vi "ObtainObject.vi"(8 "ErrorIn":errorcluster, 9 "Label":string, 10 "ObjectName":string, 11 "Type":refnum<class "ITAFObject.lvclass">) -> (0 "ErrorOut":errorcluster, 3 "ObjectOut":refnum<class "ITAFObject.lvclass">)   [LabVIEW 2021]
uses:
  Interface_TAF_ITAFObject/ITAFObject/ITAFObject.lvclass
  Interface_TAF_IApplicationConfiguration/IApplicationConfiguration/IApplicationConfiguration.lvclass
  56a36cc8-d42a-406d-9e1b-e03f28116498.vi
  <vilib>/TriekselSoft/TracerLibrary/TracerLibrary/Tracer/protected/SendMessage.vi
  <vilib>/TriekselSoft/TracerLibrary/TracerLibrary/Tracer/protected/Timestamp.vi
  56a36cc8-d42a-406d-9e1b-e03f28116498.vi/f75db090-0877-4668-94fb-75c2140b1617.vi
  <vilib>/TriekselSoft/TracerLibrary/TracerLibrary/Tracer/Tracer_Level-Debug.vi
  <vilib>/JDP Science/JSONtext/Variant to JSON Text.vi
  <vilib>/TriekselSoft/TracerLibrary/TracerLibrary/Tracer/protected/Tracer_ClassAttributes.vi
  <vilib>/JDP Science/JSONtext/LVClass Serializer/JSONtext LVClass Serializer.lvclass
  Application.lvclass/Application.ctl
  Application.lvclass
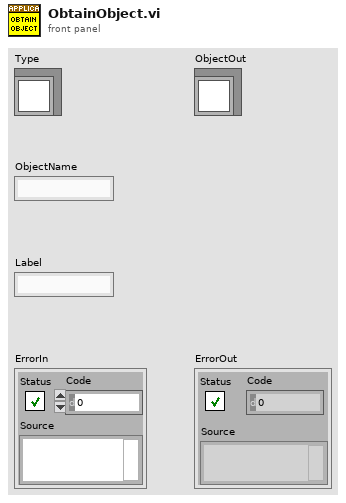
[diagram p1: front panel]
types:
  T1 = cluster{"Label":string, "ObjectName":string, "class name":string}
  T2 = typedef "Application.lvclass/ObjectAttributes.ctl" = cluster{"Objects":variant, "BasePath":path, "Application":refnum<class "Application.lvclass">}
  T3 = typedef "IApplicationConfiguration.lvclass/ObjectData.ctl" = cluster{"Label":string, "ObjectName":string, "Type":string}
  T4 = typedef "IApplicationConfiguration.lvclass/ObjectDataDetails.ctl" = cluster{"ObjectName":string, "ObjectType":string, "Interfaces":T3[]}
  T5 = typedef "ClusterArrayConversion.lvlib/BundledArray.ctl" = cluster{"Label":string, "Object":refnum<class>, "Array":bool}
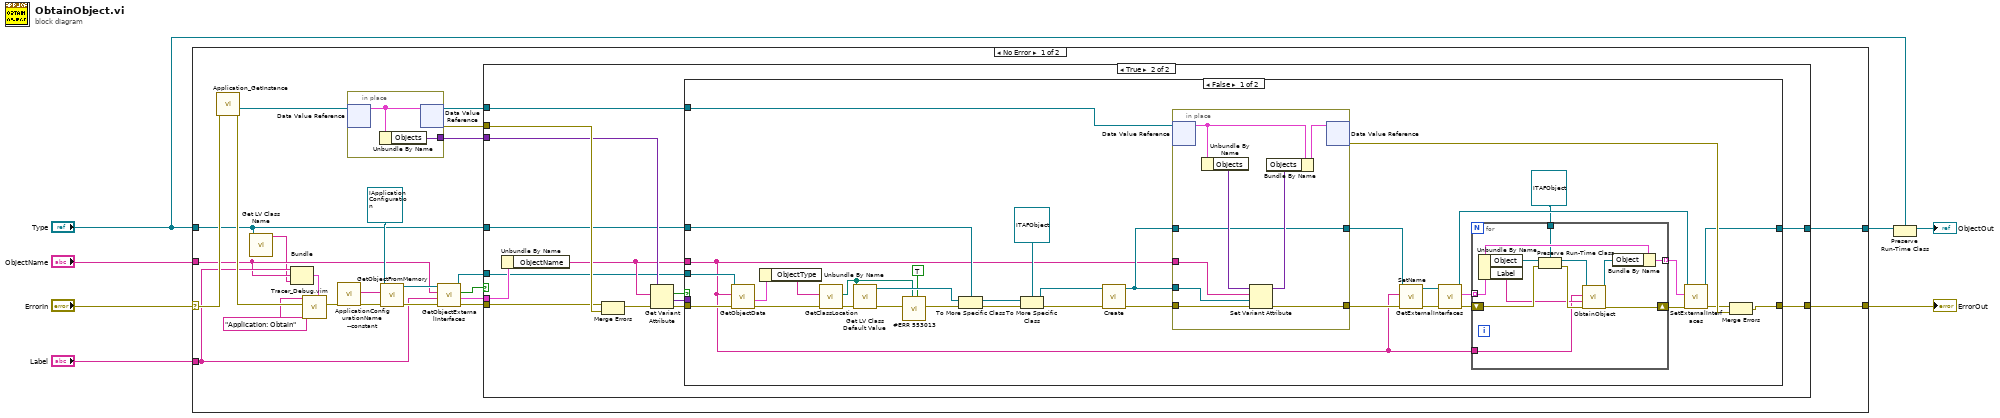
[diagram p0: block diagram]
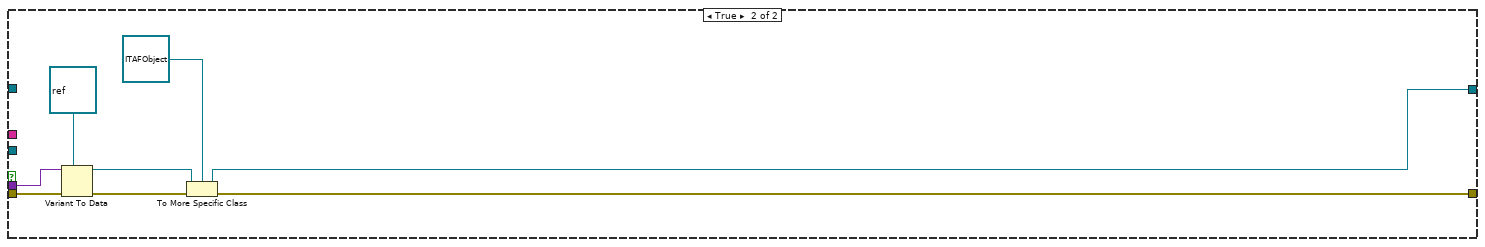
[diagram p3: hidden frame]
diagram:
  n1 = case shown="No Error" "ErrorIn" {
    selector: "ErrorIn" -> [w30 w112]
    tunnel: [w28 w112] -> w6
    tunnel: "ObjectName" -> [w13 _]
    tunnel: "Type" -> [w12 _]
    tunnel: [w23 _] -> w4
    tunnel: "Label" -> [w14 _]
    frame No Error {
      n2 = call "Application_GetInstance.vi"("ErrorIn"=w30) -> ("ErrorOut"=w25:errorcluster, "DVRRefOut"=w22:refnum<data-value>)  [unwired: 6 in, 3 out]
      n3 = call <vilib>:"Get LV Class Name.vi"("object"=w12) -> ("class name"=w11:string)  [unwired: 9 in, 1 out]
      n4 = Bundle("Label"=w14, "ObjectName"=w13, "class name"=w11) -> (w10:T1)  [unwired: 1 in]
      n5 = call "Tracer_Debug.vim"("Data"=w10, "Error In"=w25, "Text"="Application: Obtain") -> ("Error Out"=w24:errorcluster)  [unwired: 8 in]
      n6 = call "ApplicationConfigurationName --constant.vi"() -> ("AppConfigName"=w18:string)  [unwired: 10 in, 1 out]
      n7 = in-place {
        in-place-border: [w110] -> w21
        n8 = in-place-dvr #1(w22) -> (w111:T2)  [unwired: 1 out]
        n9 = Unbundle By Name(w111) -> ("Objects"=w110:variant)
        n10 = in-place-dvr #1(w111) -> (w20:refnum<data-value>, w29:errorcluster)
      }
      n11 = call "GetObjectFromMemory.vi"("ErrorIn"=w24, "ObjectName"=w18, "Type"=refnum<class "IApplicationConfiguration.lvclass"> refnum ("IApplicationStructure")) -> ("ErrorOut"=w27:errorcluster, "ObjectOut"=w17:refnum<class "IApplicationConfiguration.lvclass">)  [unwired: 7 in]
      n12 = call-dynamic "GetObjectExternalInterfaces.vi"("ErrorIn"=w27, "Label"=w14, "ThisObject"=w13, "ObjectIn"=w17) -> ("ErrorOut"=w26:errorcluster, "ObjectData"=w16:T3, "Valid"=w9:bool, "ObjectOut"=w8:refnum<class "IApplicationConfiguration.lvclass">)  [unwired: 4 in]
      n13 = case shown="True" w9 {
        tunnel: [w31 w41] -> w23
        tunnel: w29 -> [_ w46]
        tunnel: w21 -> [_ w38]
        tunnel: w20 -> [_ w37]
        tunnel: [w32 w43] -> w28
        tunnel: w26 -> [w32 w42]
        tunnel: w16 -> [_ w36]
        tunnel: w12 -> [w31 w34]
        tunnel: w8 -> [_ w33]
        frame False {
        }
        frame True {
          n14 = Unbundle By Name(w36) -> ("ObjectName"=w35:string)
          n15 = Merge Errors(w42, w46) -> (w45:errorcluster)
          n16 = Get Variant Attribute(Variant=w38, name=w35, error in=w45) -> (found=w40:bool, value=w39:variant, error out=w44:errorcluster)  [unwired: 1 in, 1 out]
          n17 = case shown="False" w40 {
            tunnel: w44 -> [w69 w109]
            tunnel: w34 -> [w61 _]
            tunnel: [w81 w107] -> w43
            tunnel: [w53 w102] -> w41
            tunnel: w39 -> [_ w105]
            tunnel: w37 -> [w66 _]
            tunnel: w35 -> [w50 _]
            tunnel: w33 -> [w51 _]
            frame False {
              n18 = call-dynamic "GetObjectData.vi"("ErrorIn"=w69, "Object"=w50, "ReferenceIn"=w51) -> ("ErrorOut"=w68:errorcluster, "Object2"=w49:T4)  [unwired: 6 in, 1 out]
              n19 = Unbundle By Name(w49) -> ("ObjectType"=w48:string)
              n20 = call "GetClassLocation.vi"("ErrorIn"=w68, "ClassString"=w48) -> ("ErrorOut"=w67:errorcluster, "ClassFilePath"=w47:path)  [unwired: 8 in]
              n21 = call <vilib>:"Get LV Class Default Value.vi"("error in (no error)"=w67, "class path"=w47) -> ("error out"=w77:errorcluster, "object"=w62:refnum<class>)  [unwired: 8 in]
              n22 = call "#ERR 553013"("MergeErrors"=TRUE, "Data"=w47, "error in (no error)"=w77) -> ("error out"=w75:errorcluster)  [unwired: 8 in]
              n23 = To More Specific Class(target class=w61, reference=w62, error in=w75) -> (specific class reference=w60:refnum<class "ITAFObject.lvclass">, error out=w76:errorcluster)
              n24 = To More Specific Class(target class=refnum<class "ITAFObject.lvclass"> refnum ("ClassActor"), reference=w60, error in=w76) -> (specific class reference=w64:refnum<class "ITAFObject.lvclass">, error out=w79:errorcluster)
              n25 = call-dynamic "Create.vi"("ErrorIn"=w79, "ObjectIn"=w64) -> ("ErrorOut"=w78:errorcluster, "ObjectOut"=w63:refnum<class "ITAFObject.lvclass">)  [unwired: 8 in]
              n26 = in-place {
                in-place-border: w63 -> [w99]
                in-place-border: w50 -> [w98]
                in-place-border: w78 -> [w101]
                in-place-border: [w100] -> w71
                in-place-border: [w93] -> w54
                in-place-border: w63 -> [w93]
                n27 = in-place-dvr #2(w66) -> (w97:T2)  [unwired: 1 out]
                n28 = Unbundle By Name(w97) -> ("Objects"=w95:variant)
                n29 = Set Variant Attribute(Variant=w95, name=w98, value=w99, error in=w101) -> (Variant out=w94:variant, error out=w100:errorcluster)  [unwired: 1 out]
                n30 = Bundle By Name(cluster=w97, "Objects"=w94) -> (w96:T2)
                n31 = in-place-dvr #2(w96) -> (w80:errorcluster)  [unwired: 1 out]
              }
              n32 = call-dynamic "SetName.vi"("ErrorIn"=w71, "Name"=w50, "ObjectIn"=w54) -> ("ErrorOut"=w74:errorcluster, "ObjectOut"=w58:refnum<class "ITAFObject.lvclass">)  [unwired: 7 in]
              n33 = call-dynamic "GetExternalInterfaces.vi"("ErrorIn"=w74, "ObjectIn"=w58) -> ("ErrorOut"=w73:errorcluster, "ExternalInterfaces"=w57:T5[], "ObjectOut"=w55:refnum<class "ITAFObject.lvclass">)  [unwired: 7 in]
              n34 = for {
                tunnel: w57 -> [w86] mode=indexing
                shift-right: [w92] -> w72
                shift-left: w73 -> [w91]
                tunnel: w50 -> [w87]
                tunnel: [w84] -> w56 mode=indexing
                tunnel: refnum<class "ITAFObject.lvclass"> refnum ("ClassActor") -> [w82]
                n35 = Unbundle By Name(w86) -> ("Object"=w89:refnum<class>, "Label"=w88:string)
                n36 = Preserve Run-Time Class(object in=w89, error in=w91, 2:w82) -> (object out=w83:refnum<class "ITAFObject.lvclass">, error out=w90:errorcluster)
                n37 = call "ObtainObject.vi"("ErrorIn"=w90, "Label"=w88, "ObjectName"=w87, "Type"=w83) -> ("ErrorOut"=w92:errorcluster, "ObjectOut"=w85:refnum<class "ITAFObject.lvclass">)  [unwired: 6 in]
                n38 = Bundle By Name(cluster=w86, "Object"=w85) -> (w84:T5)
              }
              n39 = call-dynamic "SetExternalInterfaces.vi"("ErrorIn"=w72, "ExternalInterfaces"=w56, "ObjectIn"=w55) -> ("ErrorOut"=w70:errorcluster, "ObjectOut"=w53:refnum<class "ITAFObject.lvclass">)  [unwired: 7 in]
              n40 = Merge Errors(w70, w80) -> (w81:errorcluster)
            }
            frame True {
              n41 = Variant To Data(error in=w109, type=refnum<class> refnum ("Type"), Variant=w105) -> (data=w104:refnum<class>, error out=w108:errorcluster)
              n42 = To More Specific Class(target class=refnum<class "ITAFObject.lvclass"> refnum ("ClassActor"), reference=w104, error in=w108) -> (specific class reference=w102:refnum<class "ITAFObject.lvclass">, error out=w107:errorcluster)
            }
          }
        }
      }
    }
    frame Error {
    }
  }
  "ErrorOut" <- w6
  n43 = Preserve Run-Time Class(object in=w4, 2:"Type") -> (object out=→"ObjectOut":refnum<class "ITAFObject.lvclass">)  [unwired: 1 in, 1 out]
